vi "MB Serial Master Query Write Single Register (poly).vi"(0 "VISA resource name":refnum<visa-resource-name>, 1 "Address":u16, 2 "Holding Register":u16, 4 "Timeout":u32=5000, 5 "error in":errorcluster, 6 "Serial Parameters":T1 {"Slave Address" format="%.0x"}) -> (14 "VISA resource name out":refnum<visa-resource-name>, 16 "Exception Code":u8 format="%.0x", 19 "error out":errorcluster)   [LabVIEW 2020]
doc: "The master uses this VI to write a single register to the slave. This corresponds to a public function code of 6 in the MODBUS protocol."
uses:
  <vilib>/NI Modbus.llb/MB Modbus Command.ctl
panel:
  out "Registers":cluster{"Registers":u16[], "Discrete":bool[]}
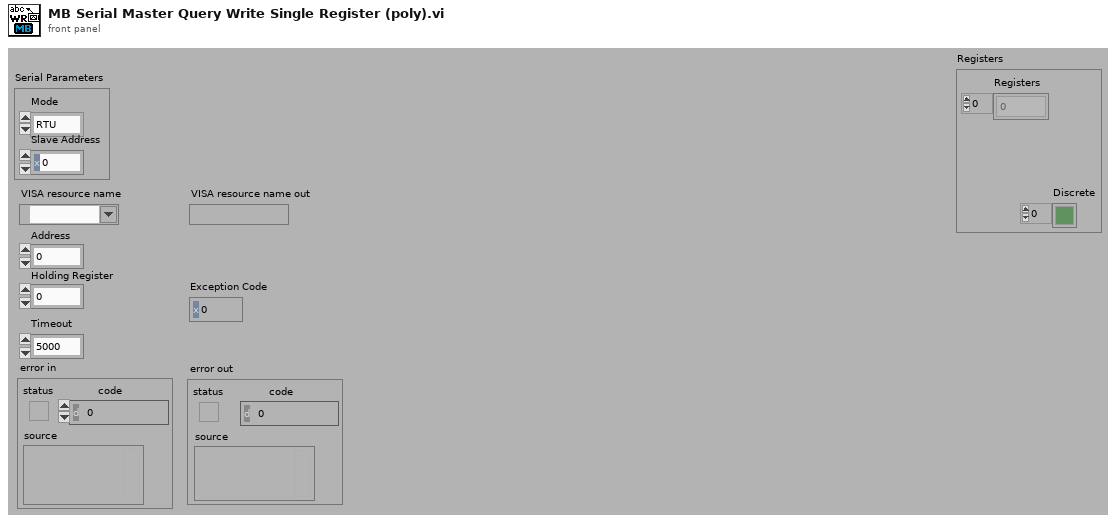
[diagram p1: front panel]
types:
  T1 = cluster{"Mode":enum16{"RTU", "ASCII"}, "Slave Address":u8}
  T2 = typedef "MB Modbus Command.ctl" = cluster{"Function Code":u8, "Starting Address":u16, "Quantity":u16, "Data":u16[], "Discrete":bool[]}
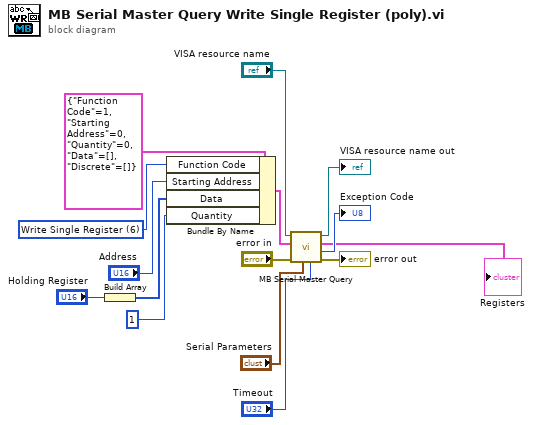
[diagram p0: block diagram]
diagram:
  w12 = u8 6 items=["Read Coils"=1, "Read Discrete Inputs"=2, "Read Holding Registers"=3, "Read Input Registers"=4, "Write Single Coil"=5, "Write Single Register"=6, "Read Exception Status"=7, "Write Multiple Coils"=15, "Write Multiple Registers"=16] ("Function Code")
  n1 = Build Array("Holding Register") -> (w4:u16[])
  n2 = Bundle By Name(cluster=T2 {"Function Code"=1, "Starting Address"=0, "Quantity"=0, "Data"=[], "Discrete"=[]} ("Modbus Command"), "Function Code"=w12, "Starting Address"="Address", "Data"=w4, "Quantity"=u16 1) -> (w13:T2)
  n3 = call <vilib>:"MB Serial Master Query.vi"("Timeout"="Timeout", "Serial Parameters"="Serial Parameters", "error in (no error)"="error in", "Modbus Command"=w13, "VISA resource name"="VISA resource name") -> ("error out"=→"error out":errorcluster, "Exception Code"=→"Exception Code":u8, "Registers"=→"Registers":cluster{"Registers":u16[], "Discrete":bool[]}, "VISA resource name out"=→"VISA resource name out":refnum<visa-resource-name>)  [unwired: 2 in, 1 out]
